vi "test_formatNumericToString_formatDoubleArrayElementToStringExistingIndex.vi"(8 "error in (no error)":errorcluster, 11 "TestCase in":refnum<class "Instrument Addon Unit Test.lvclass">) -> (0 "error out":errorcluster, 3 "TestCase out":refnum<class "Instrument Addon Unit Test.lvclass">)   [LabVIEW 2019, in "Instrument Addon Unit Test.lvclass"]
uses:
  Instrument Addon Unit Test.lvclass
  Addon/Addon Shared/Types/Metadata Channel Type.ctl
  <vilib>/addons/_JKI Toolkits/VI Tester/TestCase.llb/TestCase.lvclass
  Addon/Addon Engine/Instrument Addon Engine.lvlib
  Addon/Addon Shared/Instrument Addon Shared.lvlib
  C:/Program Files (x86)/National Instruments/LabVIEW 2019/vi.lib/addons/_JKI Toolkits/VI Tester/TestCase.llb/TestCase.lvclass
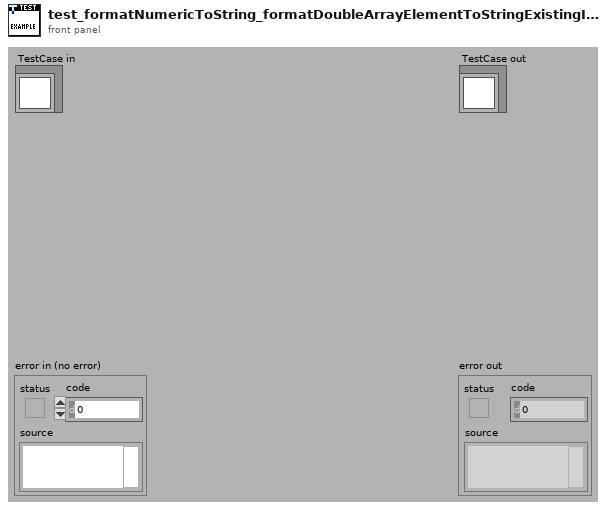
[diagram p1: front panel]
types:
  T1 = typedef "Instrument Addon Shared.lvlib/Metadata Channel Type.ctl" = enum16{"Enumerated List", "Format", "Type Cast"}
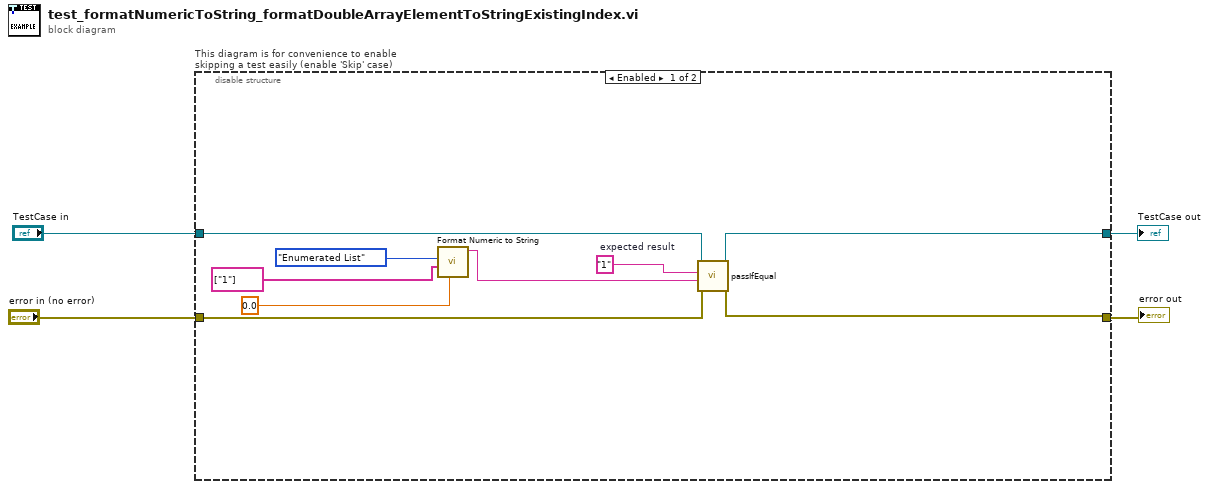
[diagram p0: block diagram]
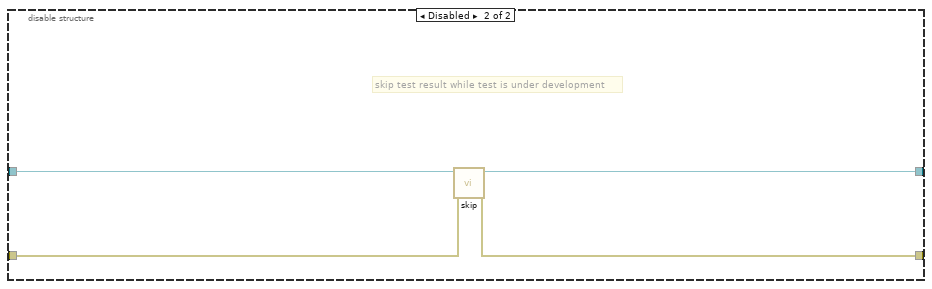
[diagram p2: hidden frame]
diagram:
  n1 = disable-structure "This diagram is for convenience to enable skipping a test easily (enable 'Skip' case)" shown="Enabled" {
    disable-tunnel: "TestCase in" -> [w12 w17]
    disable-tunnel: [w11 w15] -> w1
    disable-tunnel: [w10 w16] -> w3
    disable-tunnel: "error in (no error)" -> [w5 w14]
    frame Enabled {
      w13 = "1"  # expected result
      n2 = call "Format Numeric to String.vi"("Numeric"=0.0, "List"=string[] ["1"], "Channel Type"=Metadata_Channel_Type."Enumerated List") -> ("Value"=w6:string)  [unwired: 8 in]
      n3 = call-dynamic "passIfEqual.vi"("error in (no error)"=w5, "y"=w6, "x"=w13, "TestCase in"=w12) -> ("error out"=w10:errorcluster, "TestCase out"=w11:refnum<class "Instrument Addon Unit Test.lvclass">)  [unwired: 6 in]
    }
    frame Disabled {
      # "skip test result while test is under development"
      n4 = call <vilib>:"skip.vi"("error in (no error)"=w14, "TestCase in"=w17) -> ("error out"=w16:errorcluster, "TestCase out"=w15:refnum<class "Instrument Addon Unit Test.lvclass">)  [unwired: 8 in]
    }
  }
  "error out" <- w3
  "TestCase out" <- w1
